vi "parse_RxMessage(CommPort).vi"(11 "ReadBuffer In":u8[](array[numeric])) -> (0 "msg size":u32, 1 "error info":u32, 2 "IrigTime":T1, 3 "Message Data":u8[](array[numeric]))   [LabVIEW 2020, in "AIM664LV.lvlib"]
doc: "Parse Rx message to obtain Message Data and IRIG time."
uses:
  AIM664LV.lvlib
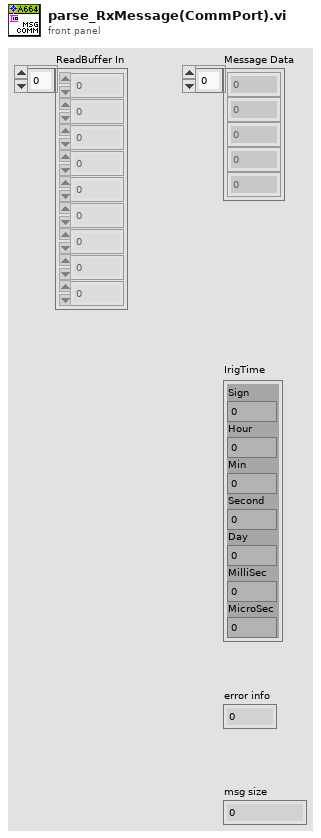
[diagram p1: front panel]
types:
  T1 = cluster{"Sign":i32, "Hour":u32, "Min":u32, "Second":u32, "Day":u32, "MilliSec":u32, "MicroSec":u32}
  T2 = typedef "AIM664LV.lvlib/IrigTime.ctl" = cluster{"Sign":i32, "Day":u32, "Hour":u32, "Min":u32, "Second":u32, "MilliSec":u32, "MicroSec":u32}
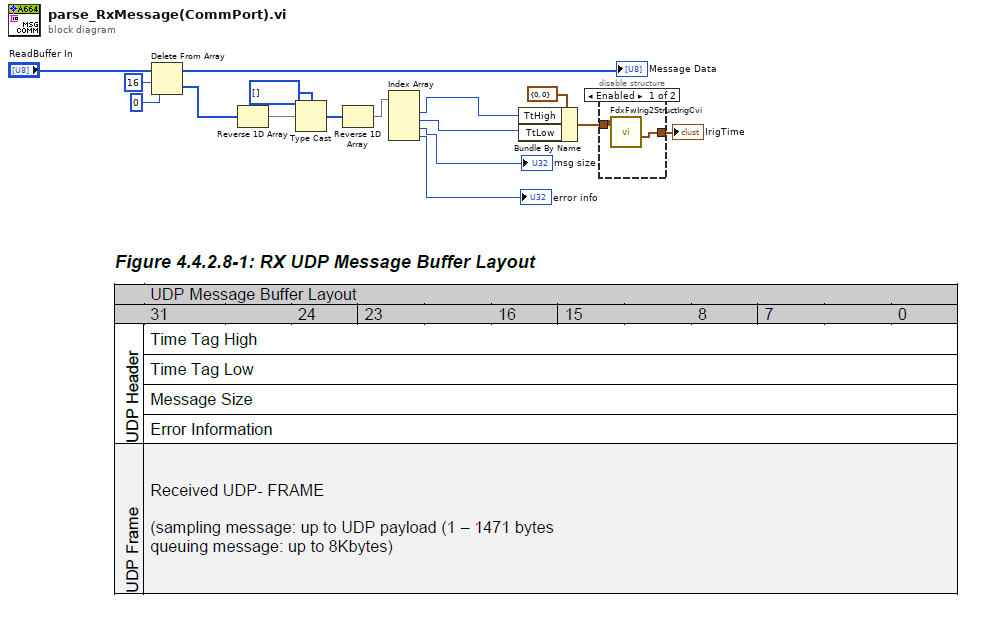
[diagram p0: block diagram]
diagram:
  n1 = Delete From Array(array="ReadBuffer In", length=16, index=0) -> (deleted portion=w9:u8[], array with subset deleted=→"Message Data":u8[])
  n2 = Reverse 1D Array(array=w9) -> (reversed array=w4:u8[])
  n3 = Type Cast(type=u32[] [] ("index"), x=w4) -> (*(type *) &x=w3:u32[])
  n4 = Reverse 1D Array(array=w3) -> (reversed array=w1:u32[])
  n5 = Index Array(array=w1) -> (element #1=w8:u32, element #2=w7:u32, element #3=→"msg size":u32, element #4=→"error info":u32)  [unwired: 4 in]
  n6 = Bundle By Name(cluster=cluster{"TtHigh":u32, "TtLow":u32} {"TtHigh"=0, "TtLow"=0} ("FwIrigTime"), "TtHigh"=w8, "TtLow"=w7) -> (w11:cluster{"TtHigh":u32, "TtLow":u32})
  n7 = disable-structure shown="Enabled" {
    disable-tunnel: w11 -> [w18 _]
    disable-tunnel: [w17 _] -> w10
    frame Enabled {
      n8 = call "FdxFwIrig2StructIrigCvi.vi"("FwIrigTime"=w18) -> ("IrigTime"=w17:T2)  [unwired: 9 in, 1 out]
    }
    frame Disabled {
    }
  }
  "IrigTime" <- w10
